vi "CSDB_Config.get config file path.vi"(5 "error in (no error)":errorcluster) -> (17 "config file path":path, 19 "error out":errorcluster)   [LabVIEW 2014, in "CSDB_Config.lvlib"]
doc: "Gets the folder where text files for configuration are stored."
uses:
  CSDB_Config.lvlib
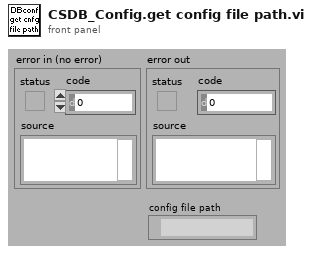
[diagram p1: front panel]
types:
  T1 = enum32{"invalid app kind", "Development System", "Run Time System", "Student Edition", "Embedded LabVIEW", "Evaluation", "Custom"}
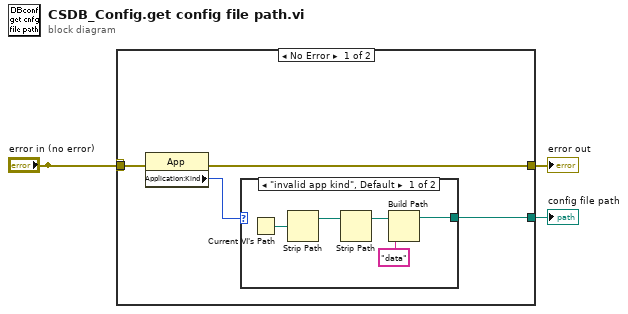
[diagram p0: block diagram]
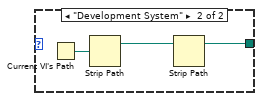
[diagram p2: hidden frame]
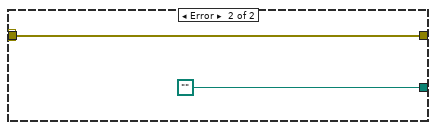
[diagram p3: hidden frame]
diagram:
  n1 = case shown="No Error" "error in (no error)" {
    selector: "error in (no error)" -> [w7 _]
    tunnel: "error in (no error)" -> [_ w17]
    tunnel: [w6 w17] -> w3
    tunnel: [w4 path ""] -> w2
    frame No Error {
      n2 = property class="App"(error in=w7) -> (error out=w6:errorcluster, "Application:Kind"=w5:T1)  [unwired: 1 in, 1 out]
      n3 = case shown="\"invalid app kind\", Default" w5 {
        tunnel: [w12 w13] -> w4
        frame "invalid app kind", Default {
          n4 = Current VI's Path() -> (path=w8:path)
          n5 = Strip Path(path=w8) -> (stripped path=w9:path)  [unwired: 1 out]
          n6 = Strip Path(path=w9) -> (stripped path=w10:path)  [unwired: 1 out]
          n7 = Build Path(base path=w10, name or relative path="data") -> (appended path=w12:path)
        }
        frame "Development System" {
          n8 = Current VI's Path() -> (path=w15:path)
          n9 = Strip Path(path=w15) -> (stripped path=w14:path)  [unwired: 1 out]
          n10 = Strip Path(path=w14) -> (stripped path=w13:path)  [unwired: 1 out]
        }
      }
    }
    frame Error {
    }
  }
  "error out" <- w3
  "config file path" <- w2
